vi "RB2 set the camera.vi"(2 "error in":errorcluster, 3 "IMAQdx Session input":T1) -> (0 "error out":errorcluster, 1 "IMAQdx Session output":T1)   [LabVIEW 2012]
doc: "This VI sets the camera values for the Point Grey Firefly camera above the pool for the Robotics II Final Project."
uses:
  <vilib>/userdefined/High Color/IMAQdx.ctl
  <resource>/objmgr/imaqdx.rc
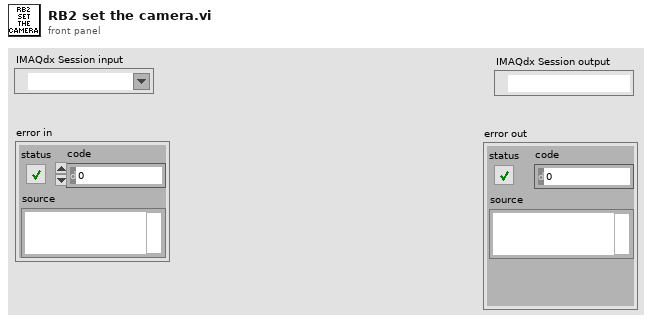
[diagram p1: front panel]
types:
  T1 = typedef "IMAQdx.ctl" = refnum<k21>
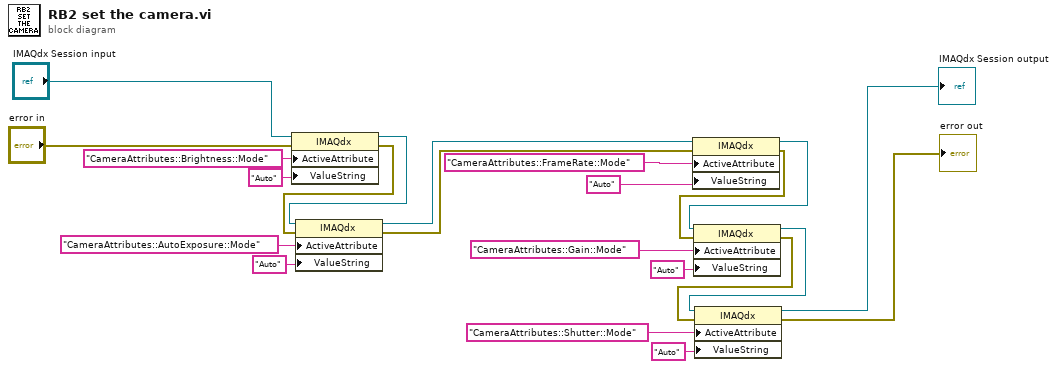
[diagram p0: block diagram]
diagram:
  n1 = property class="IMAQdx"(reference="IMAQdx Session input", error in="error in", "ActiveAttribute"="CameraAttributes::Brightness::Mode", "ValueString"="Auto") -> (reference out=w6:T1, error out=w5:errorcluster)
  n2 = property class="IMAQdx"(reference=w6, error in=w5, "ActiveAttribute"="CameraAttributes::AutoExposure::Mode", "ValueString"="Auto") -> (reference out=w2:T1, error out=w1:errorcluster)
  n3 = property class="IMAQdx"(reference=w2, error in=w1, "ActiveAttribute"="CameraAttributes::FrameRate::Mode", "ValueString"="Auto") -> (reference out=w3:T1, error out=w4:errorcluster)
  n4 = property class="IMAQdx"(reference=w3, error in=w4, "ActiveAttribute"="CameraAttributes::Gain::Mode", "ValueString"="Auto") -> (reference out=w12:T1, error out=w8:errorcluster)
  n5 = property class="IMAQdx"(reference=w12, error in=w8, "ActiveAttribute"="CameraAttributes::Shutter::Mode", "ValueString"="Auto") -> (reference out=→"IMAQdx Session output":T1, error out=→"error out":errorcluster)
